vi "Create Volatus API.vi"(8 "error in (no error)":errorcluster, 11 "Volatus Core in":refnum<class "Volatus Core.lvclass">) -> (0 "error out":errorcluster, 3 "Volatus Core out":refnum<class "Volatus Core.lvclass">)   [LabVIEW 2020, in "Volatus.lvlib" / "Volatus Core.lvclass"]
uses:
  Volatus Core.lvclass
  C:/dev/lv20CE/relink/lv-volatus/Volatus/Module/Module.lvclass
  Volatus Core.lvclass/Volatus Core.ctl
  Module/Module.lvclass/Module.ctl
  VolatusAPI/VolatusAPI.lvclass
  Module/Module.lvclass
  VolatusConfig/Node/Node.lvclass
  VolatusConfig/Cluster/Cluster.lvclass
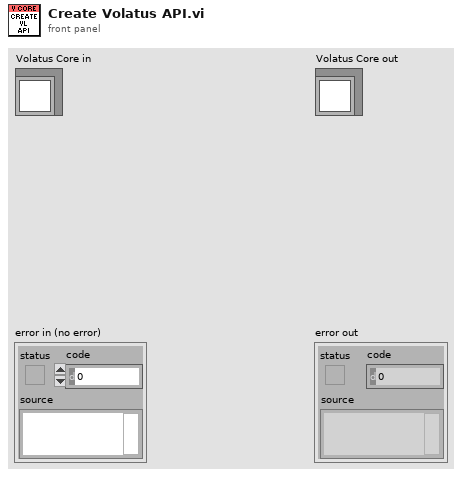
[diagram p1: front panel]
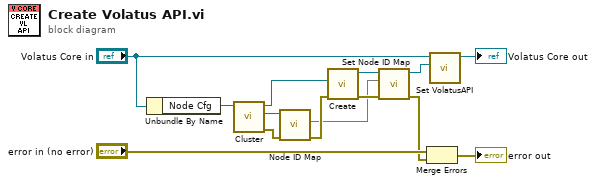
[diagram p0: block diagram]
diagram:
  n1 = Unbundle By Name("Volatus Core in") -> ("Node Cfg"=w11:refnum<class "Node.lvclass">)
  n2 = call "Cluster.vi"("Node in"=w11) -> ("error out"=w7:errorcluster, "Cluster"=w10:refnum<class "Cluster.lvclass">, "Node out"=w1:refnum<class "Node.lvclass">)  [unwired: 8 in]
  n3 = call "Node ID Map.vi"("error in (no error)"=w7, "Cluster in"=w10) -> ("error out"=w8:errorcluster, "Node ID Map"=w5:map{string, u32})  [unwired: 7 in, 1 out]
  n4 = call "Create.vi"("error in (no error)"=w8, "Node Config"=w1) -> ("error out"=w6:errorcluster, "VolatusAPI out"=w9:refnum<class "VolatusAPI.lvclass">)  [unwired: 8 in]
  n5 = call "Set Node ID Map.vi"("error in (no error)"=w6, "Node IDs"=w5, "VolatusAPI in"=w9) -> ("error out"=w2:errorcluster, "VolatusAPI out"=w4:refnum<class "VolatusAPI.lvclass">)  [unwired: 7 in]
  n6 = Merge Errors("error in (no error)", w2) -> (→"error out":errorcluster)
  n7 = call "Set VolatusAPI.vi"("VolatusAPI"=w4, "Module in"="Volatus Core in") -> ("Module out"=→"Volatus Core out":refnum<class "Volatus Core.lvclass">)  [unwired: 9 in]
